vi "AB_820_850_Project_EXE_ActiveX_Info.vi"(7 "action":T1, 8 "error in (no error)":errorcluster, 10 "activeX info in":T2, 11 "Object In":T3) -> (0 "error out":errorcluster, 2 "activeX info out":T2, 3 "Object Out":T3, 5 "empty":bool)   [LabVIEW 2020]
uses:
  <resource>/Framework/Providers/API/ItemRef.ctl
  <vilib>/AppBuilder/RW_Project/AB_RW_Project_PropBag_Action.ctl
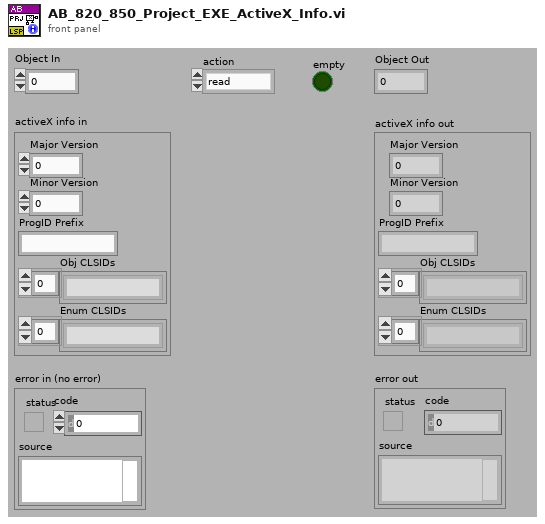
[diagram p1: front panel]
types:
  T1 = typedef "AB_RW_Project_PropBag_Action.ctl" = enum16{"read", "write", "clear", "readPrevious", "writePrevious", "clearPrevious"}
  T2 = cluster{"Major Version":u16, "Minor Version":u16, "ProgID Prefix":string, "Obj CLSIDs":string[], "Enum CLSIDs":string[]}
  T3 = typedef "ItemRef.ctl" = u64
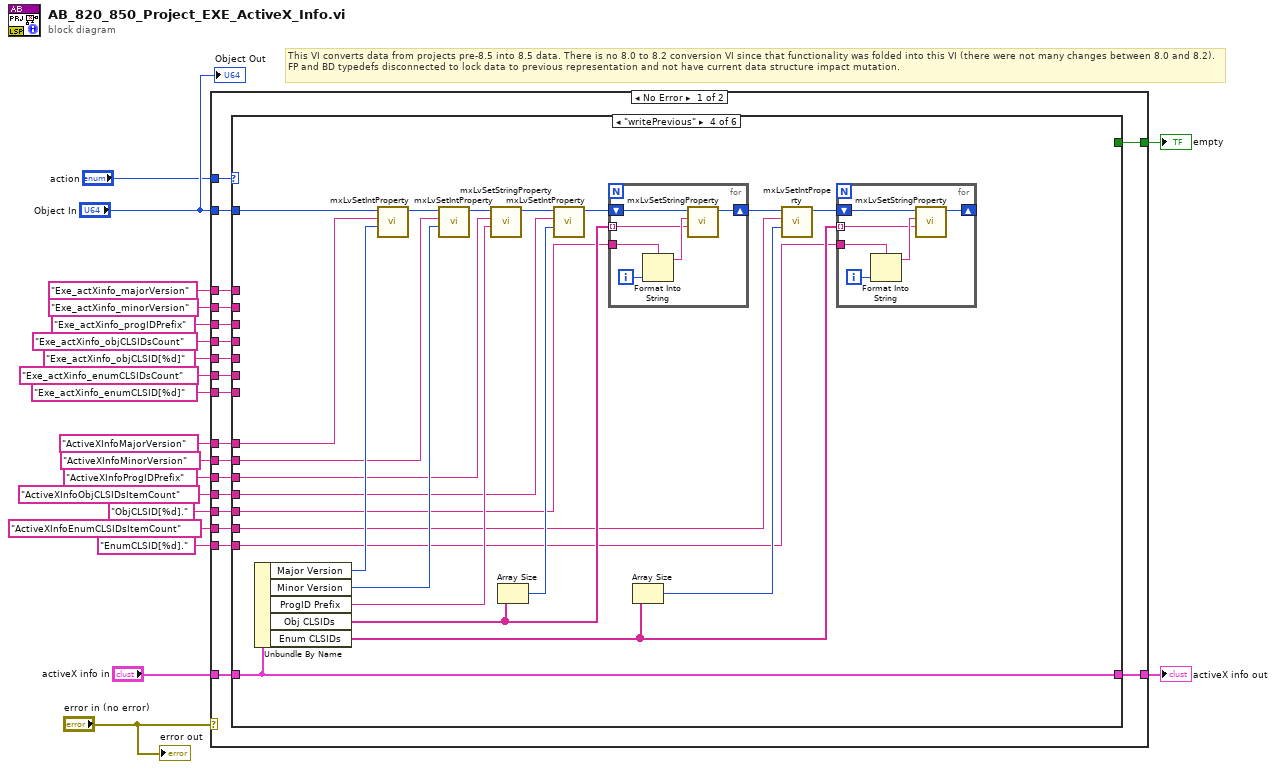
[diagram p0: block diagram]
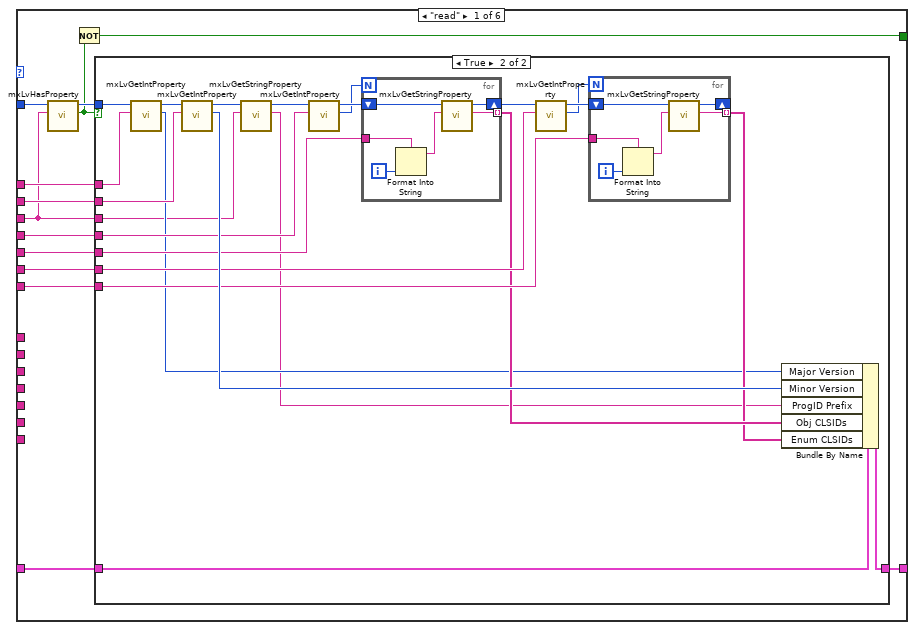
[diagram p2: hidden frame]
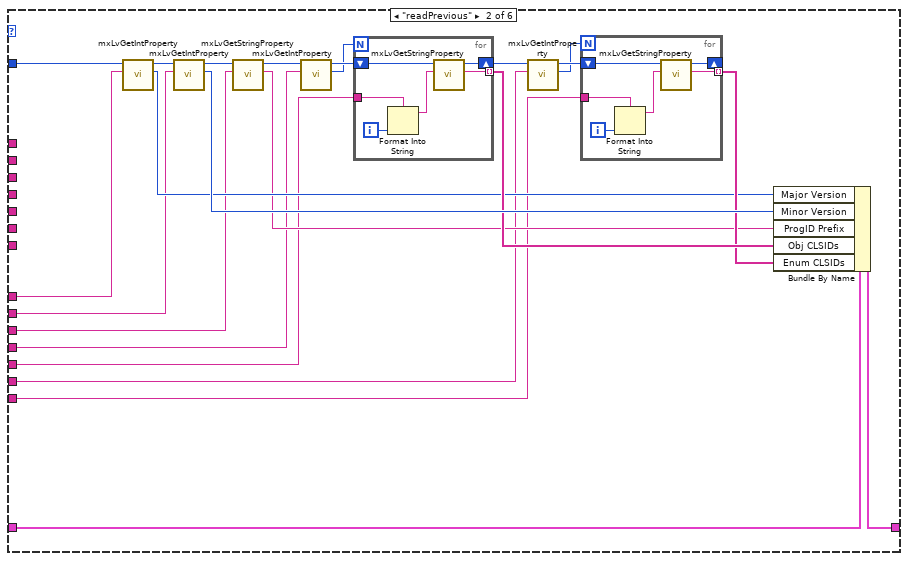
[diagram p4: hidden frame]
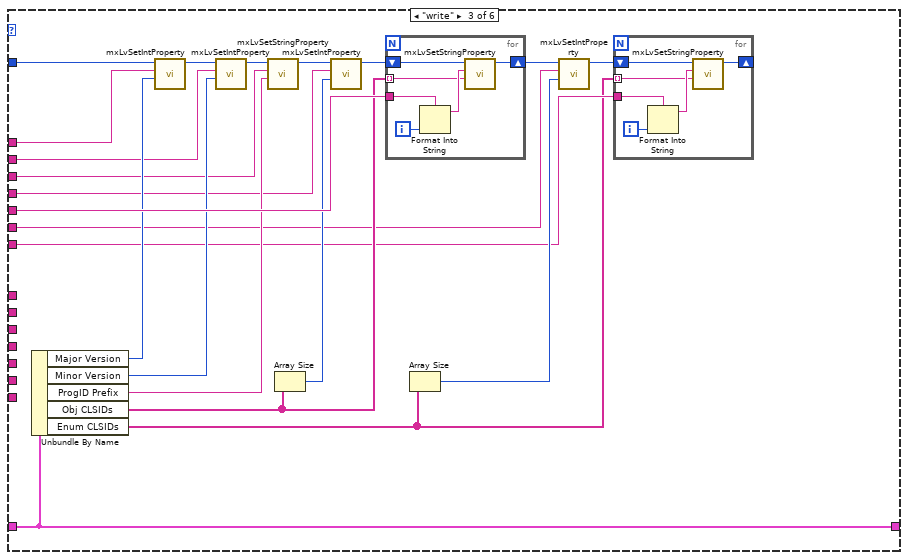
[diagram p5: hidden frame]
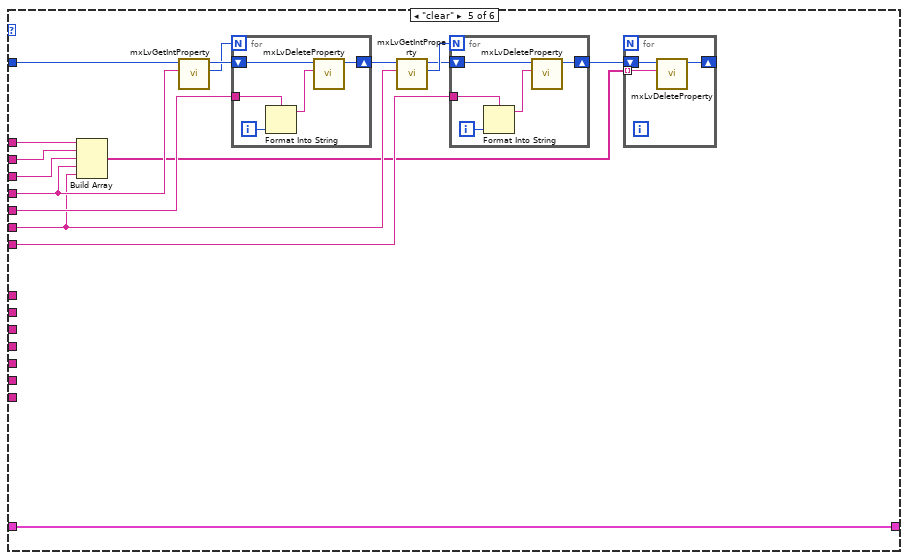
[diagram p6: hidden frame]
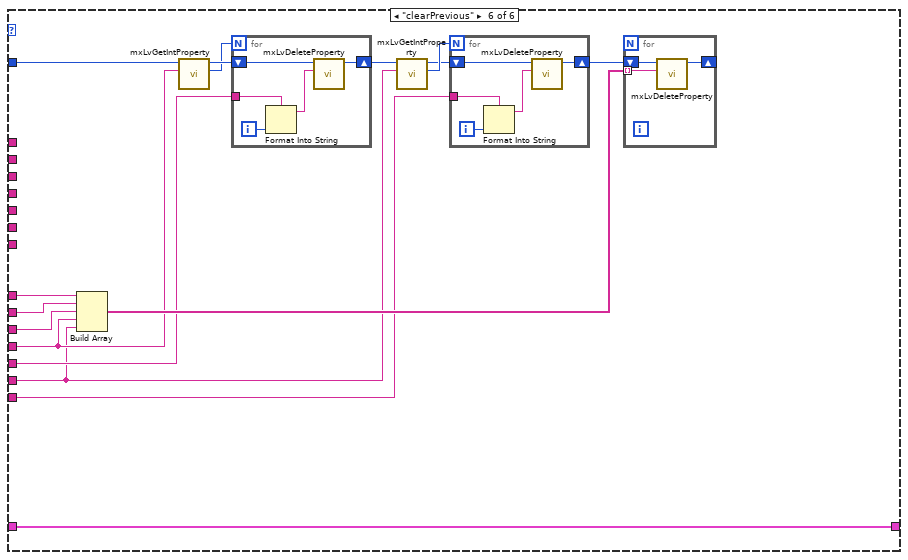
[diagram p7: hidden frame]
diagram:
  # "This VI converts data from projects pre-8.5 into 8.5 data. There is no 8.0 to 8.2 conversion VI since that functionality was folded into this VI (there were not many changes between 8.0 and 8.2).\nFP and BD typedefs disconnected to lock data to previous representation and not have current data structure impact mutation."
  n1 = case shown="No Error" "error in (no error)" {
    tunnel: "Object In" -> [w37 _]
    tunnel: [w39 _] -> w18
    tunnel: "Exe_actXinfo_majorVersion" -> [w38 _]
    tunnel: "Exe_actXinfo_minorVersion" -> [w36 _]
    tunnel: "Exe_actXinfo_progIDPrefix" -> [w35 _]
    tunnel: "activeX info in" -> [w34 _]
    tunnel: "action" -> [w33 _]
    tunnel: "Exe_actXinfo_objCLSIDsCount" -> [w32 _]
    tunnel: "Exe_actXinfo_objCLSID[%d]" -> [w31 _]
    tunnel: "Exe_actXinfo_enumCLSIDsCount" -> [w30 _]
    tunnel: "Exe_actXinfo_enumCLSID[%d]" -> [w29 _]
    tunnel: [w28 _] -> w8
    tunnel: "ActiveXInfoMajorVersion" -> [w27 _]
    tunnel: "ActiveXInfoMinorVersion" -> [w26 _]
    tunnel: "ActiveXInfoProgIDPrefix" -> [w25 _]
    tunnel: "ActiveXInfoObjCLSIDsItemCount" -> [w24 _]
    tunnel: "ObjCLSID[%d]." ("string") -> [w23 _]
    tunnel: "ActiveXInfoEnumCLSIDsItemCount" -> [w22 _]
    tunnel: "EnumCLSID[%d]." ("string") -> [w21 _]
    frame No Error {
      n2 = case shown="\"writePrevious\"" w33 {
        tunnel: [w52 w111 w142 w178 w207 w236] -> w39
        tunnel: w38 -> [w50 _ w143 _ w206 _]
        tunnel: w37 -> [w44 w96 w144 w179 w201 w233]
        tunnel: w36 -> [w49 _ w139 _ w205 _]
        tunnel: w35 -> [w42 _ w136 _ w204 _]
        tunnel: w34 -> [w51 w110 w142 w178 w207 w236]
        tunnel: w32 -> [w48 _ w133 _ w200 _]
        tunnel: w31 -> [w47 _ w145 _ w199 _]
        tunnel: w30 -> [w46 _ w126 _ w195 _]
        tunnel: w29 -> [w45 _ w125 _ w194 _]
        tunnel: [w40 _ _ _ _ _] -> w28
        tunnel: w27 -> [_ w95 _ w164 _ w227]
        tunnel: w26 -> [_ w94 _ w163 _ w226]
        tunnel: w25 -> [_ w93 _ w162 _ w225]
        tunnel: w24 -> [_ w92 _ w161 _ w224]
        tunnel: w23 -> [_ w91 _ w160 _ w223]
        tunnel: w22 -> [_ w90 _ w159 _ w222]
        tunnel: w21 -> [_ w89 _ w158 _ w221]
        frame "read" {
          n3 = call <resource>:"mxLvHasProperty.vi"("Tag"=w42, "Item"=w44) -> ("HasProperty"=w41:bool, "Item"=w43:T3)  [unwired: 7 in, 1 out]
          n4 = Not(x=w41) -> (.not. x?=w40:bool)
          n5 = case shown="True" w41 {
            tunnel: [w53 w76] -> w52
            tunnel: w51 -> [w53 w75]
            tunnel: w50 -> [_ w73]
            tunnel: w49 -> [_ w72]
            tunnel: w48 -> [_ w69]
            tunnel: w47 -> [_ w67]
            tunnel: w46 -> [_ w63]
            tunnel: w45 -> [_ w62]
            tunnel: w43 -> [_ w57]
            tunnel: w42 -> [_ w56]
            frame False {
            }
            frame True {
              n6 = call <resource>:"mxLvGetIntProperty.vi"("Tag"=w73, "Item"=w57) -> ("Value"=w59:i32, "Item"=w74:T3)  [unwired: 7 in, 1 out]
              n7 = call <resource>:"mxLvGetIntProperty.vi"("Tag"=w72, "Item"=w74) -> ("Value"=w70:i32, "Item"=w71:T3)  [unwired: 7 in, 1 out]
              n8 = call <resource>:"mxLvGetStringProperty.vi"("Tag"=w56, "Item"=w71) -> ("Value"=w58:string, "Item"=w68:T3)  [unwired: 7 in, 1 out]
              n9 = call <resource>:"mxLvGetIntProperty.vi"("Tag"=w69, "Item"=w68) -> ("Value"=w55:i32, "Item"=w66:T3)  [unwired: 7 in, 1 out]
              n10 = for {
                N: w55 -> [_]
                tunnel: w67 -> [w88]
                shift-right: [w85] -> w64
                shift-left: w66 -> [w86]
                tunnel: [w83] -> w61 mode=indexing
                i -> [w87]
                n11 = Format Into String(format string=w88, w87) -> (resulting string=w84:string)  [unwired: 2 in, 1 out]
                n12 = call <resource>:"mxLvGetStringProperty.vi"("Tag"=w84, "Item"=w86) -> ("Value"=w83:string, "Item"=w85:T3)  [unwired: 7 in, 1 out]
              }
              n13 = call <resource>:"mxLvGetIntProperty.vi"("Tag"=w63, "Item"=w64) -> ("Value"=w54:i32, "Item"=w65:T3)  [unwired: 7 in, 1 out]
              n14 = for {
                N: w54 -> [_]
                tunnel: w62 -> [w82]
                shift-right: [w79] -> _
                shift-left: w65 -> [w80]
                tunnel: [w77] -> w60 mode=indexing
                i -> [w81]
                n15 = Format Into String(format string=w82, w81) -> (resulting string=w78:string)  [unwired: 2 in, 1 out]
                n16 = call <resource>:"mxLvGetStringProperty.vi"("Tag"=w78, "Item"=w80) -> ("Value"=w77:string, "Item"=w79:T3)  [unwired: 7 in, 1 out]
              }
              n17 = Bundle By Name(cluster=w75, "Major Version"=w59, "Minor Version"=w70, "ProgID Prefix"=w58, "Obj CLSIDs"=w61, "Enum CLSIDs"=w60) -> (w76:T2)
            }
          }
        }
        frame "readPrevious" {
          n18 = call <resource>:"mxLvGetIntProperty.vi"("Tag"=w95, "Item"=w96) -> ("Value"=w100:i32, "Item"=w109:T3)  [unwired: 7 in, 1 out]
          n19 = call <resource>:"mxLvGetIntProperty.vi"("Tag"=w94, "Item"=w109) -> ("Value"=w107:i32, "Item"=w108:T3)  [unwired: 7 in, 1 out]
          n20 = call <resource>:"mxLvGetStringProperty.vi"("Tag"=w93, "Item"=w108) -> ("Value"=w99:string, "Item"=w106:T3)  [unwired: 7 in, 1 out]
          n21 = call <resource>:"mxLvGetIntProperty.vi"("Tag"=w92, "Item"=w106) -> ("Value"=w98:i32, "Item"=w105:T3)  [unwired: 7 in, 1 out]
          n22 = for {
            N: w98 -> [_]
            tunnel: w91 -> [w123]
            shift-right: [w120] -> w103
            shift-left: w105 -> [w121]
            tunnel: [w118] -> w102 mode=indexing
            i -> [w122]
            n23 = Format Into String(format string=w123, w122) -> (resulting string=w119:string)  [unwired: 2 in, 1 out]
            n24 = call <resource>:"mxLvGetStringProperty.vi"("Tag"=w119, "Item"=w121) -> ("Value"=w118:string, "Item"=w120:T3)  [unwired: 7 in, 1 out]
          }
          n25 = call <resource>:"mxLvGetIntProperty.vi"("Tag"=w90, "Item"=w103) -> ("Value"=w97:i32, "Item"=w104:T3)  [unwired: 7 in, 1 out]
          n26 = for {
            N: w97 -> [_]
            tunnel: w89 -> [w117]
            shift-right: [w114] -> _
            shift-left: w104 -> [w115]
            tunnel: [w112] -> w101 mode=indexing
            i -> [w116]
            n27 = Format Into String(format string=w117, w116) -> (resulting string=w113:string)  [unwired: 2 in, 1 out]
            n28 = call <resource>:"mxLvGetStringProperty.vi"("Tag"=w113, "Item"=w115) -> ("Value"=w112:string, "Item"=w114:T3)  [unwired: 7 in, 1 out]
          }
          n29 = Bundle By Name(cluster=w110, "Major Version"=w100, "Minor Version"=w107, "ProgID Prefix"=w99, "Obj CLSIDs"=w102, "Enum CLSIDs"=w101) -> (w111:T2)
        }
        frame "write" {
          n30 = Unbundle By Name(w142) -> ("Major Version"=w141:u16, "Minor Version"=w138:u16, "ProgID Prefix"=w135:string, "Obj CLSIDs"=w130:string[], "Enum CLSIDs"=w124:string[])
          n31 = call <resource>:"mxLvSetIntProperty.vi"("Value (0)"=w141, "Tag"=w143, "Item"=w144) -> ("Item"=w140:T3)  [unwired: 7 in, 1 out]
          n32 = call <resource>:"mxLvSetIntProperty.vi"("Value (0)"=w138, "Tag"=w139, "Item"=w140) -> ("Item"=w137:T3)  [unwired: 7 in, 1 out]
          n33 = call <resource>:"mxLvSetStringProperty.vi"("Value (\"\")"=w135, "Tag"=w136, "Item"=w137) -> ("Item"=w134:T3)  [unwired: 7 in, 1 out]
          n34 = Array Size(array=w130) -> (size(s)=w131:i32)
          n35 = call <resource>:"mxLvSetIntProperty.vi"("Value (0)"=w131, "Tag"=w133, "Item"=w134) -> ("Item"=w132:T3)  [unwired: 7 in, 1 out]
          n36 = for {
            tunnel: w145 -> [w157]
            shift-right: [w154] -> w128
            shift-left: w132 -> [w155]
            tunnel: w130 -> [w152] mode=indexing
            i -> [w156]
            n37 = Format Into String(format string=w157, w156) -> (resulting string=w153:string)  [unwired: 2 in, 1 out]
            n38 = call <resource>:"mxLvSetStringProperty.vi"("Value (\"\")"=w152, "Tag"=w153, "Item"=w155) -> ("Item"=w154:T3)  [unwired: 7 in, 1 out]
          }
          n39 = Array Size(array=w124) -> (size(s)=w127:i32)
          n40 = call <resource>:"mxLvSetIntProperty.vi"("Value (0)"=w127, "Tag"=w126, "Item"=w128) -> ("Item"=w129:T3)  [unwired: 7 in, 1 out]
          n41 = for {
            tunnel: w125 -> [w151]
            shift-right: [w148] -> _
            shift-left: w129 -> [w149]
            tunnel: w124 -> [w146] mode=indexing
            i -> [w150]
            n42 = Format Into String(format string=w151, w150) -> (resulting string=w147:string)  [unwired: 2 in, 1 out]
            n43 = call <resource>:"mxLvSetStringProperty.vi"("Value (\"\")"=w146, "Tag"=w147, "Item"=w149) -> ("Item"=w148:T3)  [unwired: 7 in, 1 out]
          }
        }
        frame "writePrevious" {
          n44 = Unbundle By Name(w178) -> ("Major Version"=w177:u16, "Minor Version"=w175:u16, "ProgID Prefix"=w173:string, "Obj CLSIDs"=w169:string[], "Enum CLSIDs"=w165:string[])
          n45 = call <resource>:"mxLvSetIntProperty.vi"("Value (0)"=w177, "Tag"=w164, "Item"=w179) -> ("Item"=w176:T3)  [unwired: 7 in, 1 out]
          n46 = call <resource>:"mxLvSetIntProperty.vi"("Value (0)"=w175, "Tag"=w163, "Item"=w176) -> ("Item"=w174:T3)  [unwired: 7 in, 1 out]
          n47 = call <resource>:"mxLvSetStringProperty.vi"("Value (\"\")"=w173, "Tag"=w162, "Item"=w174) -> ("Item"=w172:T3)  [unwired: 7 in, 1 out]
          n48 = Array Size(array=w169) -> (size(s)=w170:i32)
          n49 = call <resource>:"mxLvSetIntProperty.vi"("Value (0)"=w170, "Tag"=w161, "Item"=w172) -> ("Item"=w171:T3)  [unwired: 7 in, 1 out]
          n50 = for {
            tunnel: w160 -> [w191]
            shift-right: [w188] -> w167
            shift-left: w171 -> [w189]
            tunnel: w169 -> [w186] mode=indexing
            i -> [w190]
            n51 = Format Into String(format string=w191, w190) -> (resulting string=w187:string)  [unwired: 2 in, 1 out]
            n52 = call <resource>:"mxLvSetStringProperty.vi"("Value (\"\")"=w186, "Tag"=w187, "Item"=w189) -> ("Item"=w188:T3)  [unwired: 7 in, 1 out]
          }
          n53 = Array Size(array=w165) -> (size(s)=w166:i32)
          n54 = call <resource>:"mxLvSetIntProperty.vi"("Value (0)"=w166, "Tag"=w159, "Item"=w167) -> ("Item"=w168:T3)  [unwired: 7 in, 1 out]
          n55 = for {
            tunnel: w158 -> [w185]
            shift-right: [w182] -> _
            shift-left: w168 -> [w183]
            tunnel: w165 -> [w180] mode=indexing
            i -> [w184]
            n56 = Format Into String(format string=w185, w184) -> (resulting string=w181:string)  [unwired: 2 in, 1 out]
            n57 = call <resource>:"mxLvSetStringProperty.vi"("Value (\"\")"=w180, "Tag"=w181, "Item"=w183) -> ("Item"=w182:T3)  [unwired: 7 in, 1 out]
          }
        }
        frame "clear" {
          n58 = Build Array(w206, w205, w204, w200, w195) -> (w193:string[])
          n59 = call <resource>:"mxLvGetIntProperty.vi"("Tag"=w200, "Item"=w201) -> ("Value"=w202:i32, "Item"=w203:T3)  [unwired: 7 in, 1 out]
          n60 = for {
            N: w202 -> [_]
            tunnel: w199 -> [w220]
            shift-right: [w217] -> w196
            shift-left: w203 -> [w218]
            i -> [w219]
            n61 = Format Into String(format string=w220, w219) -> (resulting string=w216:string)  [unwired: 2 in, 1 out]
            n62 = call <resource>:"mxLvDeleteProperty.vi"("Tag"=w216, "Item"=w218) -> ("Item"=w217:T3)  [unwired: 8 in, 1 out]
          }
          n63 = call <resource>:"mxLvGetIntProperty.vi"("Tag"=w195, "Item"=w196) -> ("Value"=w198:i32, "Item"=w197:T3)  [unwired: 7 in, 1 out]
          n64 = for {
            N: w198 -> [_]
            tunnel: w194 -> [w215]
            shift-right: [w212] -> w192
            shift-left: w197 -> [w213]
            i -> [w214]
            n65 = Format Into String(format string=w215, w214) -> (resulting string=w211:string)  [unwired: 2 in, 1 out]
            n66 = call <resource>:"mxLvDeleteProperty.vi"("Tag"=w211, "Item"=w213) -> ("Item"=w212:T3)  [unwired: 8 in, 1 out]
          }
          n67 = for {
            shift-right: [w209] -> _
            shift-left: w192 -> [w210]
            tunnel: w193 -> [w208] mode=indexing
            n68 = call <resource>:"mxLvDeleteProperty.vi"("Tag"=w208, "Item"=w210) -> ("Item"=w209:T3)  [unwired: 8 in, 1 out]
          }
        }
        frame "clearPrevious" {
          n69 = Build Array(w227, w226, w225, w224, w222) -> (w229:string[])
          n70 = call <resource>:"mxLvGetIntProperty.vi"("Tag"=w224, "Item"=w233) -> ("Value"=w234:i32, "Item"=w235:T3)  [unwired: 7 in, 1 out]
          n71 = for {
            N: w234 -> [_]
            tunnel: w223 -> [w249]
            shift-right: [w246] -> w230
            shift-left: w235 -> [w247]
            i -> [w248]
            n72 = Format Into String(format string=w249, w248) -> (resulting string=w245:string)  [unwired: 2 in, 1 out]
            n73 = call <resource>:"mxLvDeleteProperty.vi"("Tag"=w245, "Item"=w247) -> ("Item"=w246:T3)  [unwired: 8 in, 1 out]
          }
          n74 = call <resource>:"mxLvGetIntProperty.vi"("Tag"=w222, "Item"=w230) -> ("Value"=w232:i32, "Item"=w231:T3)  [unwired: 7 in, 1 out]
          n75 = for {
            N: w232 -> [_]
            tunnel: w221 -> [w244]
            shift-right: [w241] -> w228
            shift-left: w231 -> [w242]
            i -> [w243]
            n76 = Format Into String(format string=w244, w243) -> (resulting string=w240:string)  [unwired: 2 in, 1 out]
            n77 = call <resource>:"mxLvDeleteProperty.vi"("Tag"=w240, "Item"=w242) -> ("Item"=w241:T3)  [unwired: 8 in, 1 out]
          }
          n78 = for {
            shift-right: [w238] -> _
            shift-left: w228 -> [w239]
            tunnel: w229 -> [w237] mode=indexing
            n79 = call <resource>:"mxLvDeleteProperty.vi"("Tag"=w237, "Item"=w239) -> ("Item"=w238:T3)  [unwired: 8 in, 1 out]
          }
        }
      }
    }
    frame Error {
    }
  }
  "activeX info out" <- w18
  "empty" <- w8
  "Object Out" <- "Object In"
  "error out" <- "error in (no error)"
